vi "SeparateChannelTypes.vi"(11 "All Channels":string[](array[string])) -> (2 "Vib Channels":string[](array[string]), 3 "Temperature Channels":string[](array[string]))   [LabVIEW 2017]
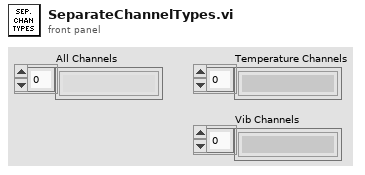
[diagram p1: front panel]
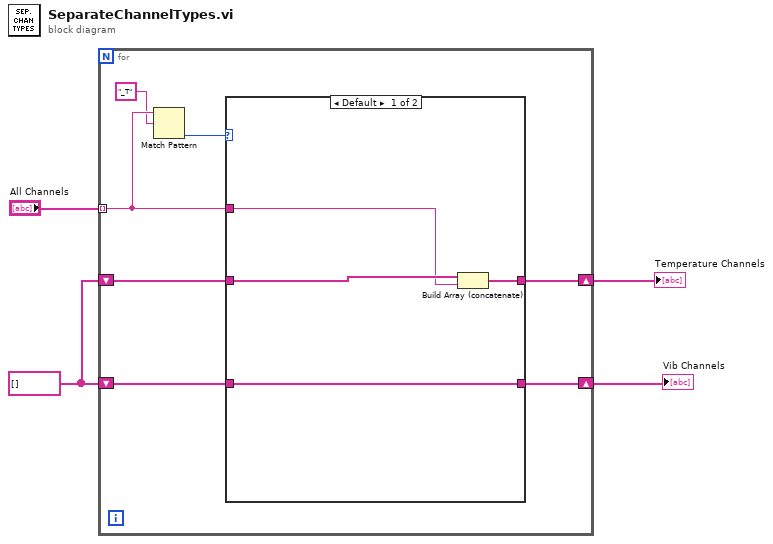
[diagram p0: block diagram]
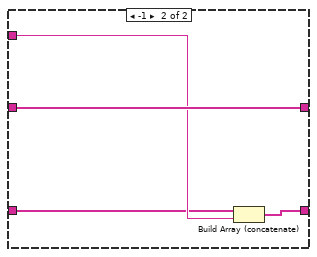
[diagram p2: hidden frame]
diagram:
  w2 = string[] []
  n1 = for {
    tunnel: "All Channels" -> [w10] mode=indexing
    shift-right: [w8] -> w1
    shift-left: w2 -> [w7]
    shift-right: [w6] -> w3
    shift-left: w2 -> [w5]
    n2 = Match Pattern(string=w10, regular expression="_T") -> (offset past match=w11:i32)  [unwired: 1 in, 3 out]
    n3 = case shown="Default" w11 {
      tunnel: w10 -> [w12 w18]
      tunnel: [w15 w19] -> w8
      tunnel: w7 -> [w13 w19]
      tunnel: [w14 w17] -> w6
      tunnel: w5 -> [w14 w16]
      frame Default {
        n4 = Build Array (concatenate)(w13, w12) -> (w15:string[])
      }
      frame -1 {
        n5 = Build Array (concatenate)(w16, w18) -> (w17:string[])
      }
    }
  }
  "Temperature Channels" <- w1
  "Vib Channels" <- w3
